vi "Get Common Path.vi"(8 "error in":errorcluster, 10 "relative path of LVLIB folders":path[](array[path]), 11 "custom device path":path) -> (0 "error out":errorcluster, 3 "common path":path)   [LabVIEW 2020, in "Template Tool.lvlib"]
uses:
  Template Tool.lvlib
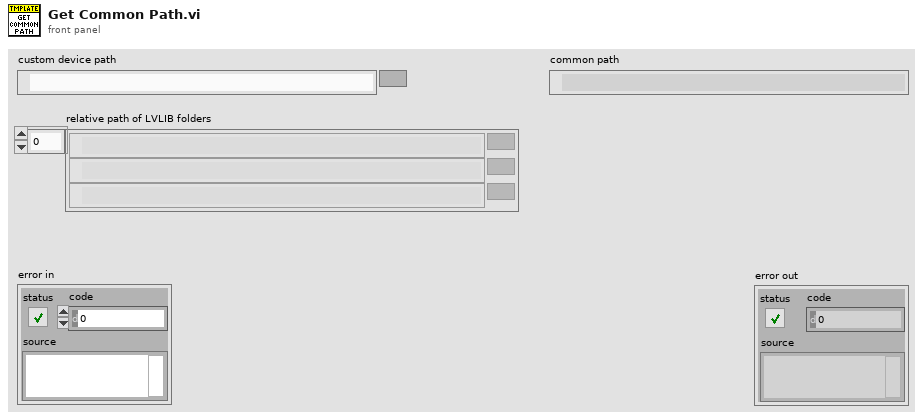
[diagram p1: front panel]
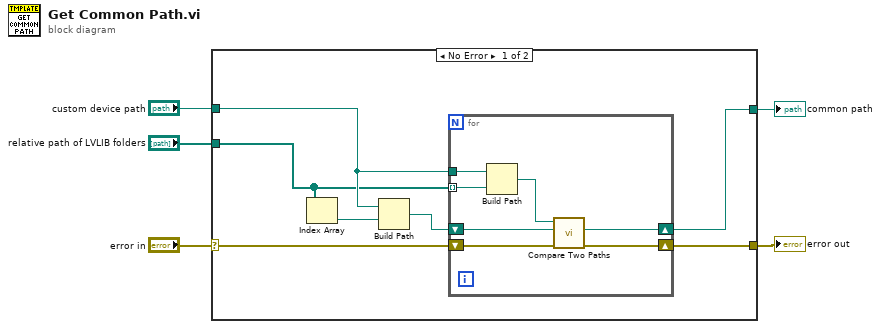
[diagram p0: block diagram]
diagram:
  n1 = case shown="No Error" "error in" {
    selector: "error in" -> [w8 w20]
    tunnel: "custom device path" -> [w10 _]
    tunnel: [w7 w20] -> w4
    tunnel: [w6 _] -> w3
    tunnel: "relative path of LVLIB folders" -> [w9 _]
    frame No Error {
      n2 = Index Array(array=w9) -> (element=w11:path)  [unwired: 1 in]
      n3 = Build Path(base path=w10, name or relative path=w11) -> (appended path=w12:path)
      n4 = for {
        tunnel: w9 -> [w18] mode=indexing
        shift-right: [w19] -> w6
        shift-left: w12 -> [w15]
        tunnel: w10 -> [w16]
        shift-right: [w13] -> w7
        shift-left: w8 -> [w14]
        n5 = Build Path(base path=w16, name or relative path=w18) -> (appended path=w17:path)
        n6 = call <vilib>:"Compare Two Paths.vi"("error in (no error)"=w14, "Path 2"=w15, "Path 1"=w17) -> ("error out"=w13:errorcluster, "Common Path"=w19:path)  [unwired: 5 in, 2 out]
      }
    }
    frame Error {
    }
  }
  "error out" <- w4
  "common path" <- w3
